vi "Zero Finder.vi"(4 "array":dbl[](array[numeric])) -> (1 "fractional zeros":dbl[](array[numeric]))   [LabVIEW 2013]
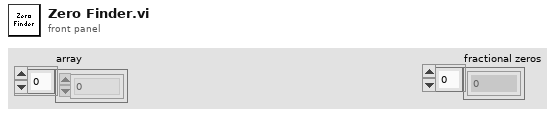
[diagram p1: front panel]
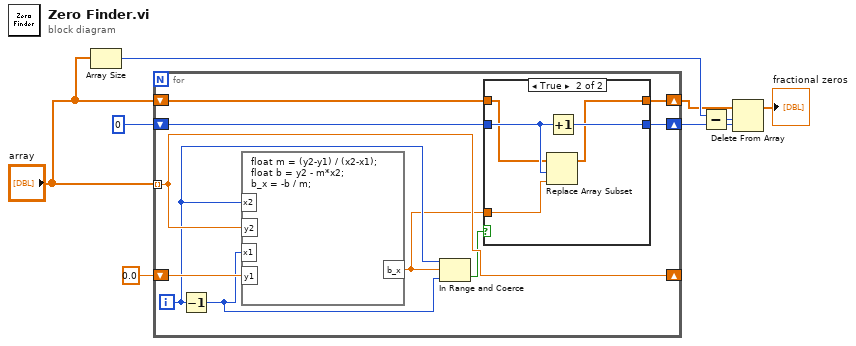
[diagram p0: block diagram]
diagram:
  n1 = Array Size(array="array") -> (size(s)=w4:i32)
  n2 = for {
    shift-right: [w17] -> _
    shift-left: 0.0 -> [w18]
    tunnel: "array" -> [w17] mode=indexing
    shift-right: [w11] -> w2
    shift-left: 0 -> [w12]
    shift-right: [w9] -> w3
    shift-left: "array" -> [w10]
    i -> [w15]
    n3 = Decrement(x=w15) -> (x-1=w16:i32)
    n4 = formula code="float m = (y2-y1) / (x2-x1);\nfloat b = y2 - m*x2;\nb_x = -b / m;"("x2"=w15, "y2"=w17, "x1"=w16, "y1"=w18) -> ("b_x"=w13:dbl)
    n5 = In Range and Coerce(upper limit=w15, x=w13, lower limit=w16) -> (In Range?=w14:bool)  [unwired: 1 out]
    n6 = case shown="True" w14 {
      tunnel: w13 -> [_ w23]
      tunnel: w12 -> [w20 w24]
      tunnel: [w20 w25] -> w11
      tunnel: w10 -> [w19 w21]
      tunnel: [w19 w22] -> w9
      frame False {
      }
      frame True {
        n7 = Replace Array Subset(array=w21, new element=w23, index=w24) -> (w22:dbl[])
        n8 = Increment(x=w24) -> (x+1=w25:i32)
      }
    }
  }
  n9 = Subtract(x=w4, y=w2) -> (x-y=w5:i32)
  n10 = Delete From Array(array=w3, length=w5, index=w2) -> (array with subset deleted=→"fractional zeros":dbl[])  [unwired: 1 out]
